vi "Expt 11.vi"() -> ()   [LabVIEW 2020]
panel:
  out "Fibonacci":i32[](array[numeric])
  in  "Amplitude":dbl
  in  "Numeric":i32
  out "current time":timestamp
  in  "stop":bool
  out "Sine Wave":dbl(graph)
  in  "Frequency (w)":dbl(slide) scale=0.0..10.0
  # "1)"
  # "2)"
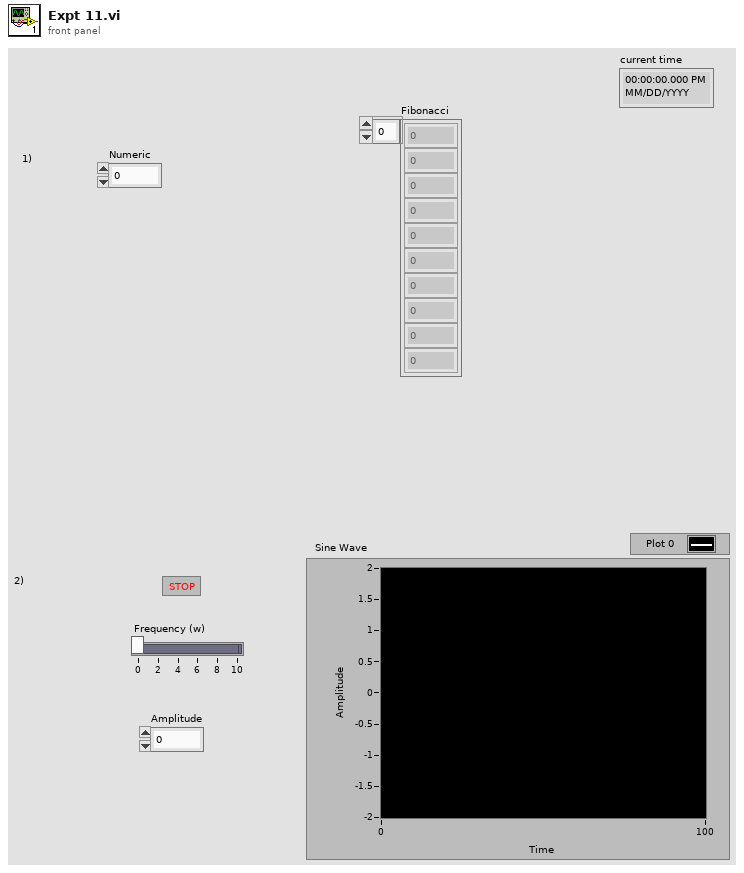
[diagram p1: front panel]
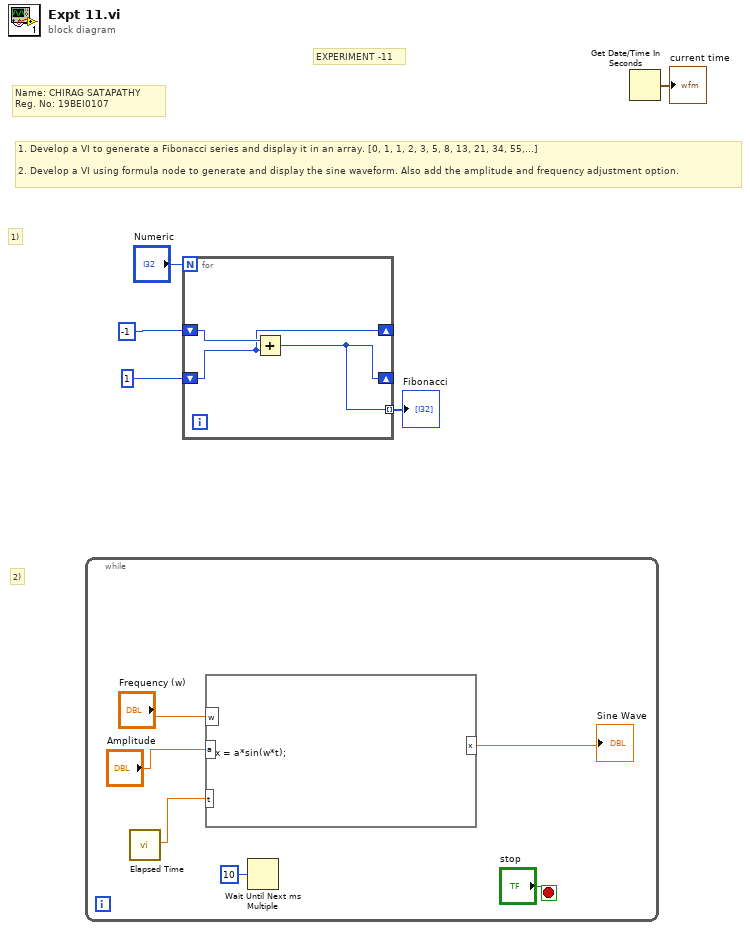
[diagram p0: block diagram]
diagram:
  # "1)"
  # "2)"
  # "1. Develop a VI to generate a Fibonacci series and display it in an array. [0, 1, 1, 2, 3, 5, 8, 13, 21, 34, 55,…]\n\n2. Develop a VI using formula node to generate and display the sine waveform. Also add the amplitude and frequency adjustment option."
  # "Name: CHIRAG SATAPATHY\nReg. No: 19BEI0107"
  # "EXPERIMENT -11"
  n1 = while {
    stop <- "stop" stop-if-true
    n2 = call "Elapsed Time"() -> ("Elapsed Time (s)"=w8:dbl)  [unwired: 12 in, 7 out]
    n3 = formula code="x = a*sin(w*t);"("w"="Frequency (w)", "t"=w8, "a"="Amplitude") -> ("x"=→"Sine Wave":dbl)
    n4 = Wait Until Next ms Multiple(millisecond multiple=u32 10) -> ()  [unwired: 1 out]
  }
  n5 = for {
    N: "Numeric" -> [_]
    shift-right: [w13] -> _
    shift-left: -1 -> [w14]
    shift-right: [w12] -> _
    shift-left: 1 -> [w13]
    tunnel: [w12] -> w1 mode=indexing
    n6 = Add(x=w14, y=w13) -> (x+y=w12:i32)
  }
  "Fibonacci" <- w1
  n7 = Get Date/Time In Seconds() -> (seconds since 1Jan1904=→"current time":timestamp)
